vi "NumericOps3.vi"() -> ()   [LabVIEW 2019]
panel:
  out "Pi":dbl=3.141592653589793
  out "x*y":dbl
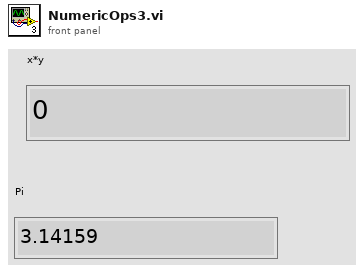
[diagram p1: front panel]
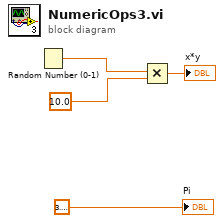
[diagram p0: block diagram]
diagram:
  n1 = Random Number (0-1)() -> (number: 0 to 1=w4:dbl)
  n2 = Multiply(x=w4, y=10.0) -> (x*y=→"x*y":dbl)
  "Pi" <- 3.141592653589793
